vi "ReadReal.vi"(10 "Offset":u32, 11 "Data":string) -> (2 "OffsetOut":u32, 3 "Value":sgl)   [LabVIEW 2012]
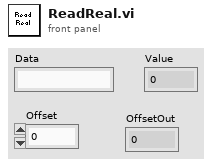
[diagram p1: front panel]
types:
  T1 = enum16{"big-endian, network order", "native, host order", "little-endian"}
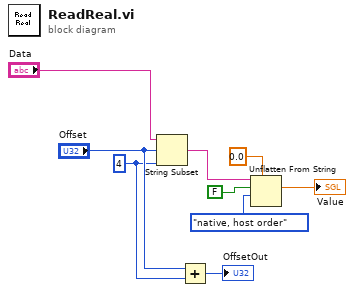
[diagram p0: block diagram]
diagram:
  w2 = 4 ("length (rest)")
  n1 = String Subset(string="Data", offset (0)="Offset", length (rest)=w2) -> (substring=w5:string)
  n2 = Add(x="Offset", y=w2) -> (x+y=→"OffsetOut":u32)
  n3 = Unflatten From String(type=sgl 0.0 ("length (rest)"), binary string=w5, data includes array or string size? (T)=FALSE, byte order (0:big-endian, network order)=T1."native, host order") -> (value=→"Value":sgl)  [unwired: 1 in, 2 out]
